vi "test_std_roll.vi"() -> ()   [LabVIEW 2020]
uses:
  <vilib>/Utility/tdmsutil.llb/TDMS Generate Random Data (U8).vi
panel:
  out "Waveform Graph":u8[](graph)
  in  "Array":dbl[](array[numeric])
  out "x <= y? 2":bool
  in  "Std range":i32
  in  "stop":bool
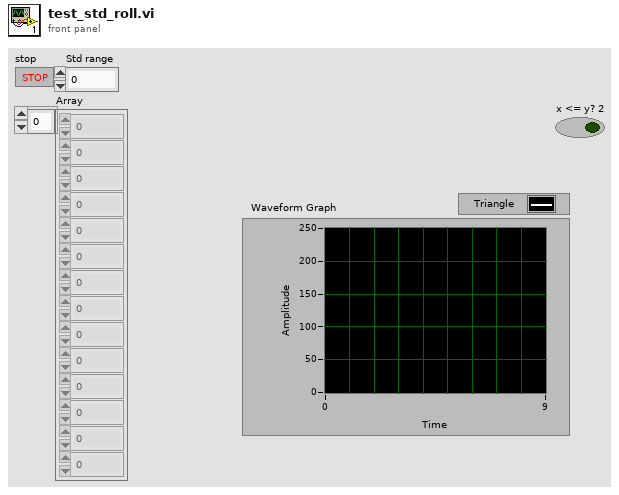
[diagram p1: front panel]
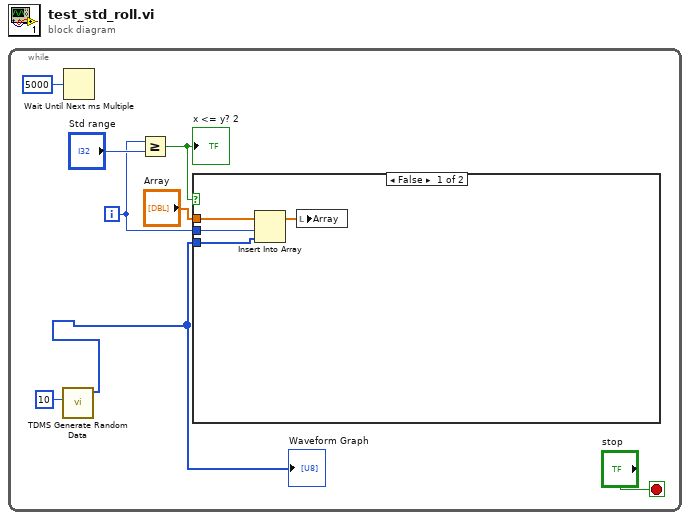
[diagram p0: block diagram]
diagram:
  n1 = while {
    i -> [w5]
    stop <- "stop" stop-if-true
    n2 = call-poly <vilib>:"TDMS Generate Random Data.vi"("number of samples"=u32 10) -> ("data"=w2:u8[])  [unwired: 9 in, 1 out]
    "Waveform Graph" <- w2
    n3 = Wait Until Next ms Multiple(millisecond multiple=u32 5000) -> ()  [unwired: 1 out]
    n4 = Greater Or Equal?(x=w5, y="Std range") -> (x >= y?=w7:bool)
    "x <= y? 2" <- w7
    n5 = case shown="False" w7 {
      tunnel: w2 -> [w11 _]
      tunnel: w5 -> [w12 _]
      tunnel: "Array" -> [w9 _]
      frame False {
        n6 = Insert Into Array(array=w9, index=w12, new element=w11) -> (w10:dbl[])
        n7 = local write "Array"(w10) -> ()
      }
      frame True {
      }
    }
  }
